vi "2dnonlinear lev-mar fit.vi"(5 "Standard Deviation":dbl[](array[numeric]) format="%.2f", 8 "max iteration":i32=200, 9 "Initial Guess Coefficients":dbl[](array[numeric]) format="%.2f", 10 "Y":dbl[](array[numeric]) format="%.2f", 11 "X":dbl[](array[numeric]) format="%.2f") -> (0 "error":i32, 1 "mse":dbl format="%.4e", 2 "Best Fit":dbl[](array[numeric]) format="%.2f", 3 "Best Fit Coefficients":dbl[](array[numeric]) format="%.2f", 4 "Covariance":dbl[][](array[numeric]) format="%.2f")   [LabVIEW 2009]
doc: "NonLinear Lev-Mar Fit:\n==================\n\nThis VI uses the Levenberg-Marquardt algorithm to determine the least squares set of coefficients that best fit the set of input data points(X,Y) as expressed by a nonlinear function y=f(x,a) where a is the set of coefficients. This VI also gives the best fit curve y=f(x.a). \n\nThe user needs to open a sub-VI \"Target Fnc & Deriv NonLin\" and inputs his/her nonlinear function f(x,a) in the Formula Node. If the user choose formula caculation for derivative method, he/she needs to input the partial deriative of f(x,a) with respect to a as well. \n\nInputs:\nX: experiment data points.\nY: experiment data points.\nStandard Deviation: standard deviation of each experiment data.If you don't have knowledge about this parameter, just leave it empty.\nInitial Guess Coefficients: Your guessed coefficients. If this is too far from the appropriate coefficients, the VI maybe will fail to return the appropriate coeficients and best fit curve.\nmax iteration: max iteration the algrothim will try. If it can not converge when it reaches the max iteration. The VI will return an error.\nderivative: There are two ways to caculate the partial derivative of f(x,a) with respect to coefficients a. If you choose nemerical caculation, the VI will use numerical method to caculate them internally. If you choose formula caculation, you need to input the derivative formula in the subvi Target Fnc & Deriv NonLin. formula caculation is more precise than numerical caculation.\n\nOutputs:\nBest Guess Coefficients: the least squares coefficients.\nBest Fit: the best fit curve f(x,a).\nCovariance: covariance matrix of Best Guess Coefficients.\nmse: mse=1/n*sum[(y(i)-f(x(i),a))/std(i)]^2)\n (std: Standard Deviation)"
uses:
  <vilib>/Analysis/baseanly.llb/Real Inverse Matrix.vi
  <vilib>/Analysis/NI_AALBase.lvlib
panel:
  # "Array Nonlinear  Lev-Mar  Fit"
  # "Modified by Christian Altenbach to allow fitting of arrays. \ncaltenba@ucla.edu"
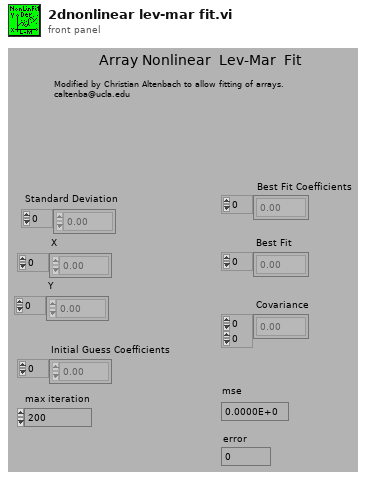
[diagram p1: front panel]
types:
  T1 = typedef "NI_Matrix.lvlib/RealMatrix.ctl" = dbl[][]
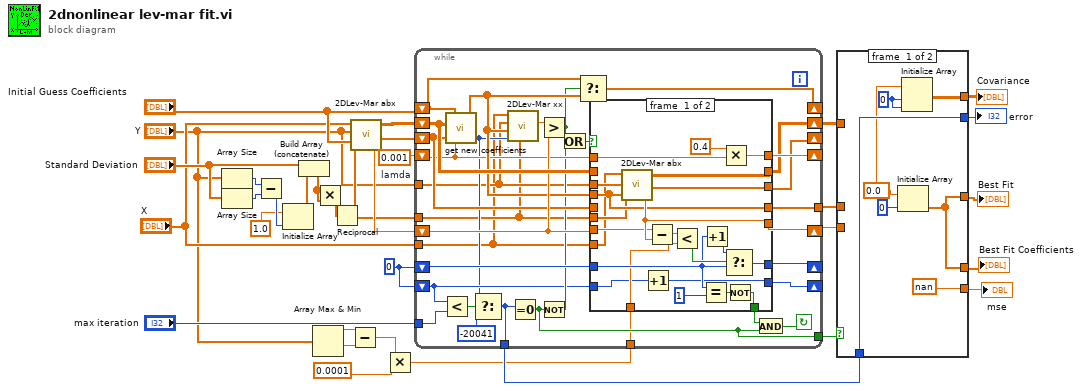
[diagram p0: block diagram]
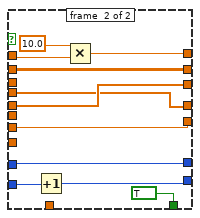
[diagram p2: hidden frame]
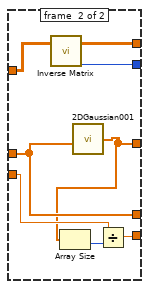
[diagram p3: hidden frame]
diagram:
  w24 = 0
  w32 = 0.001  # lamda
  n1 = Array Size(array="Y") -> (size(s)=w13:i32)
  n2 = Array Size(array="Standard Deviation") -> (size(s)=w14:i32)
  n3 = Subtract(x=w13, y=w14) -> (x-y=w15:i32)
  n4 = Initialize Array(1.0, w15) -> (w16:dbl[])
  n5 = Build Array (concatenate)("Standard Deviation", w16) -> (w9:dbl[])
  n6 = Array Max & Min(array="Y") -> (max value=w8:dbl, min value=w7:dbl)  [unwired: 2 out]
  n7 = Multiply(x=w9, y=w9) -> (x*y=w11:dbl[])
  n8 = Reciprocal(x=w11) -> (1/x=w10:dbl[])
  n9 = Subtract(x=w8, y=w7) -> (x-y=w6:dbl)
  n10 = call "2DLev-Mar abx.vi"("X"="X", "Y"="Y", "Coefficients"="Initial Guess Coefficients", "W"=w10) -> ("Alpha"=w33:dbl[][], "Beta"=w31:dbl[], "chiSqr"=w30:dbl)  [unwired: 2 in]
  n11 = Multiply(x=w6, y=0.0001) -> (x*y=w5:dbl)
  n12 = while {
    shift-right: [w64] -> _
    shift-left: w32 -> [w53]
    shift-right: [w63] -> _
    shift-left: "Initial Guess Coefficients" -> [w36]
    shift-right: [w62] -> w18
    shift-left: w33 -> [w61]
    shift-right: [w60] -> _
    shift-left: w31 -> [w55]
    shift-right: [w59] -> w29
    shift-left: w30 -> [w58]
    shift-right: [w56] -> _
    shift-left: w24 -> [w57]
    tunnel: [w52] -> w28
    tunnel: [w49] -> w25
    tunnel: w5 -> [w48]
    shift-right: [w44] -> _
    shift-left: w24 -> [w43]
    tunnel: "max iteration" -> [w39]
    tunnel: [w38] -> w19
    tunnel: "Y" -> [w37]
    tunnel: w10 -> [w35]
    tunnel: "X" -> [w34]
    stop <- w51 continue-if-true
    n13 = Less?(x=w43, y=w39) -> (x < y?=w42:bool)
    n14 = call "get new coefficients.vi"("lamda"=w53, "Beta"=w55, "Alpha"=w61, "Coefficients"=w36) -> ("error"=w40:i32, "New Coefficients"=w54:dbl[])
    n15 = Select(t=w40, s=w42, f=-20041) -> (s? t:f=w38:i32)
    n16 = call "2DLev-Mar xx.vi"("W"=w35, "error"=w40, "Coefficients"=w54, "Y"=w37, "X"=w34) -> ("chiSqr"=w65:dbl)  [unwired: 1 in]
    n17 = Equal To 0?(x=w38) -> (x = 0?=w49:bool)
    n18 = Greater?(x=w65, y=w58) -> (0:w46:bool)
    n19 = Not(x=w49) -> (.not. x?=w45:bool)
    n20 = Or(x=w46, y=w45) -> (x .or. y?=w47:bool)
    n21 = Select(t=w36, s=w46, f=w54) -> (s? t:f=w63:dbl[])
    n22 = case shown="False" w47 {
      tunnel: w53 -> [w86 w97]
      tunnel: [w85 w96] -> w64
      tunnel: [w84 w95] -> w62
      tunnel: w61 -> [_ w95]
      tunnel: [w83 w91] -> w60
      tunnel: [w82 w94] -> w59
      tunnel: w58 -> [w81 w94]
      tunnel: w57 -> [w76 w93]
      tunnel: [w77 w93] -> w56
      tunnel: [w73 TRUE] -> w50
      tunnel: w54 -> [w70 w90]
      tunnel: w55 -> [_ w91]
      tunnel: [w70 w90] -> w52
      tunnel: w48 -> [w72 _]
      tunnel: [w69 w89] -> w44
      tunnel: w43 -> [w71 w88]
      tunnel: w37 -> [w68 _]
      tunnel: w35 -> [w67 _]
      tunnel: w34 -> [w66 _]
      frame #0 {
        n23 = call "2DLev-Mar abx.vi"("X"=w66, "Y"=w68, "Coefficients"=w70, "W"=w67) -> ("Alpha"=w84:dbl[][], "Beta"=w83:dbl[], "chiSqr"=w82:dbl)  [unwired: 2 in]
        n24 = Increment(x=w71) -> (x+1=w69:i32)
        n25 = Subtract(x=w81, y=w82) -> (x-y=w80:dbl)
        n26 = Less?(x=w80, y=w72) -> (x < y?=w79:bool)
        n27 = Equal?(x=w76, y=1) -> (x = y?=w74:bool)
        n28 = Increment(x=w76) -> (x+1=w78:i32)
        n29 = Multiply(x=0.4, y=w86) -> (x*y=w85:dbl)
        n30 = Select(t=w78, s=w79, f=w76) -> (s? t:f=w77:i32)
        n31 = Not(x=w74) -> (.not. x?=w73:bool)
      }
      frame #1 {
        n32 = Increment(x=w88) -> (x+1=w89:i32)
        n33 = Multiply(x=10.0, y=w97) -> (x*y=w96:dbl)
      }
    }
    n34 = And(x=w50, y=w49) -> (x .and. y?=w51:bool)
  }
  n35 = case shown="True" w25 {
    tunnel: w28 -> [_ w107]
    tunnel: [w103 w107] -> w27
    tunnel: [nan w113] -> w26
    tunnel: [w103 w106] -> w1
    tunnel: w29 -> [_ w111]
    tunnel: [w101 w110] -> w21
    tunnel: [w100 w109] -> w20
    tunnel: w19 -> [w100 _]
    tunnel: w18 -> [_ w108]
    frame #0 {
      w99 = 0.0 ("Element Data")
      w102 = 0
      n36 = Initialize Array(w99, 0) -> (w103:dbl[])
      n37 = Initialize Array(w99, w102, w102) -> (w101:dbl[][])
    }
    frame #1 {
      n38 = call-poly <vilib>:"Inverse Matrix.vi"("Input Matrix"=w108) -> ("error"=w109:i32, "Inverse Matrix"=w110:T1)  [unwired: 1 in]
      n39 = call "2DGaussian001.vi"("Paramters"=w107) -> ("Flattened Image"=w106:dbl[])
      n40 = Array Size(array=w106) -> (size(s)=w112:i32)
      n41 = Divide(x=w111, y=w112) -> (x/y=w113:dbl)
    }
  }
  "mse" <- w26
  "Best Fit Coefficients" <- w27
  "Best Fit" <- w1
  "error" <- w20
  "Covariance" <- w21
